vi "ztscopeM Acquisition Query.vi"(8 "error in":errorcluster, 11 "Instrument Handle In":i32) -> (0 "error out":errorcluster, 1 "Acquire Count":i32, 2 "Acquire Type":i32, 3 "Instrument Handle Out":i32, 4 "Initiate Continuously":i32, 5 "Trigger Mode":i32)   [LabVIEW 2013]
doc: "Query the acquisition settings of the oscilloscope."
uses:
  ztscopeM.dll
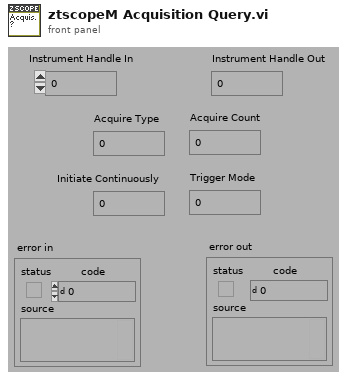
[diagram p1: front panel]
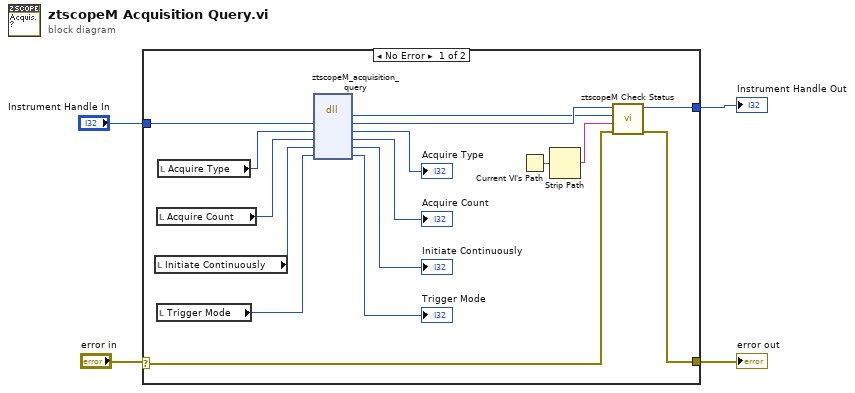
[diagram p0: block diagram]
diagram:
  n1 = case shown="No Error" "error in" {
    selector: "error in" -> [w7 w22]
    tunnel: [w6 w22] -> w1
    tunnel: "Instrument Handle In" -> [w20 w21]
    tunnel: [w5 w21] -> w3
    frame No Error {
      n2 = local read "Initiate Continuously"() -> (w15:i32)
      n3 = local read "Acquire Count"() -> (w17:i32)
      n4 = local read "Trigger Mode"() -> (w13:i32)
      n5 = local read "Acquire Type"() -> (w19:i32)
      n6 = dll-call lib="C:/Program Files/National Instruments/instr.lib/ztscopem/ztscopeM.dll" fn="ztscopeM_acquisition_query"("instrumentHandle"=w20, "acquireType"=w19, "acquireCount"=w17, "initiateContinuously"=w15, "triggerMode"=w13) -> (w8:i32, "instrumentHandle"=w9:i32, "acquireType"=→"Acquire Type":i32, "acquireCount"=→"Acquire Count":i32, "initiateContinuously"=→"Initiate Continuously":i32, "triggerMode"=→"Trigger Mode":i32)  [unwired: 3 in, 2 out]
      n7 = Current VI's Path() -> (path=w11:path)
      n8 = Strip Path(path=w11) -> (name=w10:string)  [unwired: 1 out]
      n9 = call "ztscopeM Check Status.vi"("error in"=w7, "name of VI"=w10, "status"=w8, "instrument handle in"=w9) -> ("error out"=w6:errorcluster, "instrument handle out"=w5:i32)  [unwired: 2 in]
    }
    frame Error {
    }
  }
  "Instrument Handle Out" <- w3
  "error out" <- w1
